vi "LEBITVacuum.CreateServicesAndEvent.vi"(0 "i ref in":refnum<vi>, 5 "error in(no error)":errorcluster) -> (14 "i ref out":refnum<vi>, 19 "error out":errorcluster)   [LabVIEW 2014, in "LEBITVacuum.lvlib"]
doc: "This is the constructor of a class.\n\nLicense Agreement for this software:\n\nCopyright (C)\nGesellschaft für Schwerionenforschung, GSI\nPlanckstr. 1\n64291 Darmstadt\nGermany\n\nContact: D.Beck@gsi.de \n\nThis program is free software; you can redistribute it and/or modify it under the terms of the \nGNU General Public License as published by the Free Software Foundation; either version 2 of \nthe license, or (at your option) any later version.\n\nThis program is distributed in the hope that it will be useful, but WITHOUT ANY WARRANTY; \nwithout even the implied warranty of MERCHANTABILITY or FITNESS FOR A PARTICULAR PURPOSE. See the GNU General License for more details (http://www.gnu.org).\n\nGesellschaft für Schwerionenforschung, GSI\nPlanckstr. 1, 64291 Darmstadt, Germany\nFor all questions and ideas contact: M.Richter@gsi.de, H.Brand@gsi.de or D.Beck@gsi.de.\nLast update: 16-JUN-2004"
uses:
  LEBITVacuum.lvlib
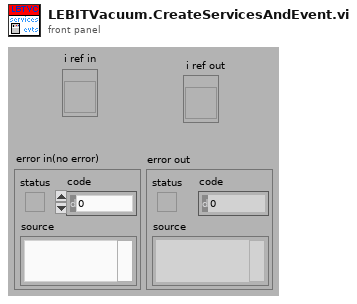
[diagram p1: front panel]
types:
  T1 = typedef "LEBITVacuum.lvlib/LEBITVacuum.i attribute.ctl" = cluster{"setValuePLC":string[], "nickNames":string[], "setValuePLCServiceID":i32[], "monValuePLC":string[], "SetValueServiceID":i32[], "MonValueServiceID":i32[], "SetValue":i16[], "AllPLCValues":string[], "CondSpecial2DArray":string[][], "CondSpecialIndex":i32[], "ReasonForLocking":string, "ReasonForLockingID":i32, "enableValuePLC":string[], "OverwriteCloseSafetyPLC":string[], "OverwriteOpenSafetyPLC":string[], "OverwriteCloseSafetyPLCServiceID":i32[], "OverwriteOpenSafetyPLCServiceID":i32[], "MKS Address Array":i32[][], "MKS MeasurementServiceID":i32[], "MKS Measurement":string[], "CRYO Measurement":string[][], "CRYO MeasurementServiceID":i32[], "Special":string[], "Start Date":string, "MKS VISA resource":refnum<visa-resource-name>, "CRYO VISA resource":refnum<visa-resource-name>}
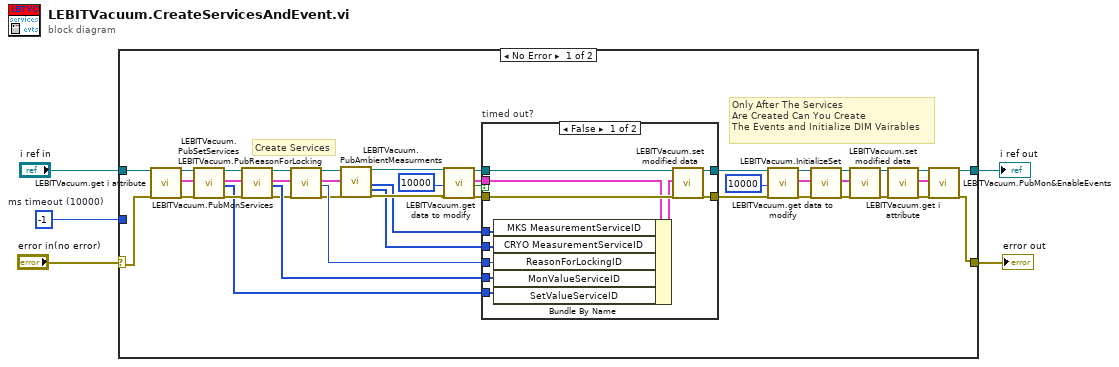
[diagram p0: block diagram]
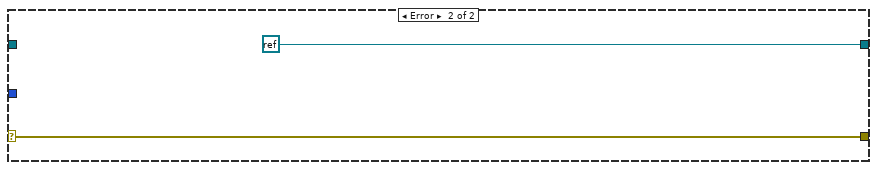
[diagram p3: hidden frame]
diagram:
  w1 = -1  # ms timeout (10000)
  n1 = case shown="No Error" "error in(no error)" {
    selector: "error in(no error)" -> [w46 w62]
    tunnel: [w7 w62] -> w5
    tunnel: "i ref in" -> [w47 _]
    tunnel: [w6 refnum<k0> refnum] -> w2
    tunnel: w1 -> [_ _]
    frame No Error {
      # "Create Services"
      # "Only After The Services\nAre Created Can You Create\nThe Events and Initialize DIM Vairables"
      n2 = call "LEBITVacuum.get i attribute.vi"("i ref in"=w47, "error in (no error)"=w46) -> ("i ref out"=w45:refnum<vi>, "i attribute"=w37:T1, "error out"=w44:errorcluster)  [unwired: 15 in]
      n3 = call "LEBITVacuum.PubSetServices.vi"("i ref in"=w45, "i attribute in"=w37, "error in"=w44) -> ("i ref out"=w43:refnum<vi>, "i attribute out"=w36:T1, "SetValueServiceID"=w34:i32[], "error out"=w42:errorcluster)  [unwired: 13 in]
      n4 = call "LEBITVacuum.PubMonServices.vi"("i ref in"=w43, "i attribute in"=w36, "error in"=w42) -> ("i ref out"=w32:refnum<vi>, "i attribute out"=w30:T1, "MonValueServiceID"=w33:i32[], "error out"=w31:errorcluster)  [unwired: 13 in]
      n5 = call "LEBITVacuum.PubReasonForLocking.vi"("i ref in"=w32, "i attribute in"=w30, "error in"=w31) -> ("i ref out"=w28:refnum<vi>, "i attribute out"=w24:T1, "my_serviceID"=w29:i32, "error out"=w25:errorcluster)  [unwired: 13 in]
      n6 = call "LEBITVacuum.PubAmbientMeasurments.vi"("i ref in"=w28, "i attribute in"=w24, "error in"=w25) -> ("i ref out"=w27:refnum<vi>, "MKS MeasurementServiceID"=w22:i32[], "CRYO MeasurementServiceID"=w23:i32[], "error out"=w26:errorcluster)  [unwired: 12 in, 1 out]
      n7 = call "LEBITVacuum.get data to modify.vi"("i ref in"=w27, "ms timeout (10000)"=10000, "error in (no error)"=w26) -> ("i ref out"=w40:refnum<vi>, "i attribute"=w38:T1, "timed out"=w41:bool, "error out"=w39:errorcluster)  [unwired: 13 in]
      n8 = case "timed out?" shown="False" w41 {
        tunnel: [w58 w60] -> w11
        tunnel: [w57 w59] -> w10
        tunnel: w40 -> [w56 w60]
        tunnel: w39 -> [w55 w59]
        tunnel: w38 -> [w54 _]
        tunnel: w34 -> [w52 _]
        tunnel: w33 -> [w51 _]
        tunnel: w29 -> [w50 _]
        tunnel: w22 -> [w49 _]
        tunnel: w23 -> [w48 _]
        frame False {
          n9 = Bundle By Name(cluster=w54, "MKS MeasurementServiceID"=w49, "CRYO MeasurementServiceID"=w48, "ReasonForLockingID"=w50, "MonValueServiceID"=w51, "SetValueServiceID"=w52) -> (w53:T1)
          n10 = call "LEBITVacuum.set modified data.vi"("i ref in"=w56, "i attribute"=w53, "error in (no error)"=w55) -> ("i ref out"=w58:refnum<vi>, "error out"=w57:errorcluster)  [unwired: 15 in]
        }
        frame True {
        }
      }
      n11 = call "LEBITVacuum.get data to modify.vi"("i ref in"=w11, "ms timeout (10000)"=10000, "error in (no error)"=w10) -> ("i ref out"=w13:refnum<vi>, "i attribute"=w17:T1, "error out"=w12:errorcluster)  [unwired: 13 in, 1 out]
      n12 = call "LEBITVacuum.InitializeSet.vi"("i ref in"=w13, "i attribute in"=w17, "error in"=w12) -> ("i ref out"=w20:refnum<vi>, "i attribute out"=w19:T1, "error out"=w18:errorcluster)  [unwired: 14 in]
      n13 = call "LEBITVacuum.set modified data.vi"("i ref in"=w20, "i attribute"=w19, "error in (no error)"=w18) -> ("i ref out"=w9:refnum<vi>, "error out"=w8:errorcluster)  [unwired: 15 in]
      n14 = call "LEBITVacuum.get i attribute.vi"("i ref in"=w9, "error in (no error)"=w8) -> ("i ref out"=w14:refnum<vi>, "i attribute"=w16:T1, "error out"=w15:errorcluster)  [unwired: 15 in]
      n15 = call "LEBITVacuum.PubMon&EnableEvents.vi"("i ref in"=w14, "i attribute in"=w16, "error in"=w15) -> ("i ref out"=w6:refnum<vi>, "error out"=w7:errorcluster)  [unwired: 14 in, 1 out]
    }
    frame Error {
    }
  }
  "i ref out" <- w2
  "error out" <- w5
